vi "DNL_INL.vi"(8 "error in (no error)":errorcluster caption="错误输入（无错误）", 11 "采集信号输入":waveform(dbl)[](array[waveform])) -> (0 "error out":errorcluster caption="错误输出", 1 "INL - Min":ext, 2 "INL - Max":ext, 3 "DNL - Min":dbl, 4 "DNL":cluster{i32, i32, "Y[i]=X[i]*a+b":dbl[]}, 5 "DNL - Max":dbl, 6 "INL":cluster{dbl, i32, ext[]}, 7 "Transfer Curve":cluster{dbl[], i32[]}[](array[cluster]))   [LabVIEW 2019]
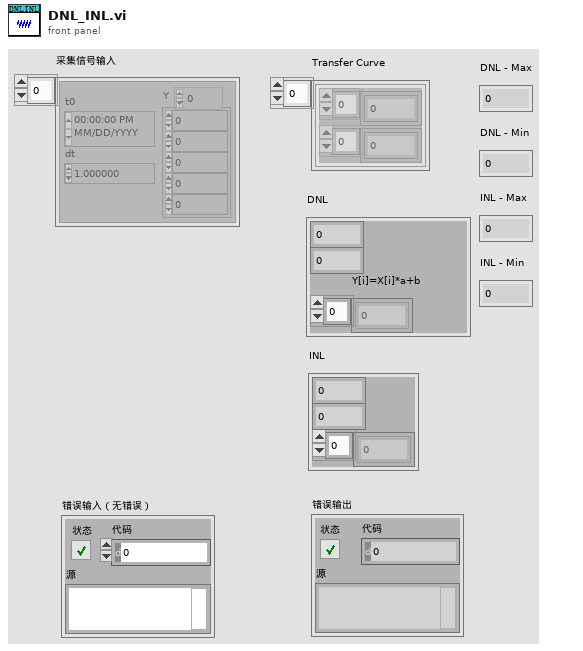
[diagram p1: front panel]
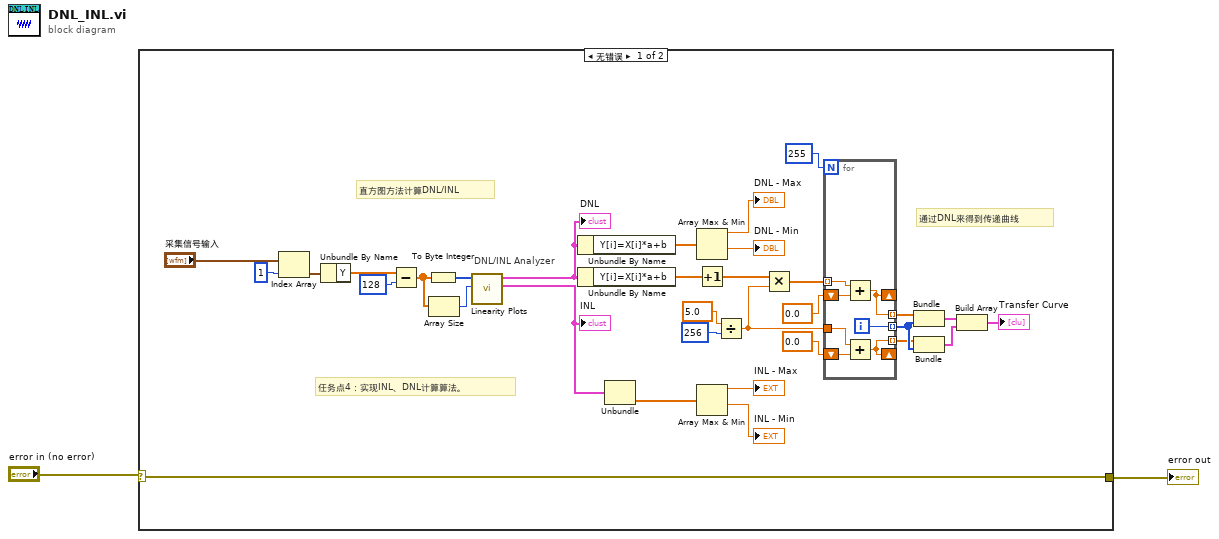
[diagram p0: block diagram]
diagram:
  n1 = case shown="无错误" "error in (no error)" {
    selector: "error in (no error)" -> [w3 w42]
    tunnel: [w3 w42] -> w1
    frame No Error {
      # "通过DNL来得到传递曲线"
      # "直方图方法计算DNL/INL"
      # "任务点4：实现INL、DNL计算算法。"
      # "DNL/INL Analyzer"
      n2 = Index Array(array="采集信号输入", index=1) -> (element=w9:waveform(dbl))
      n3 = Unbundle By Name(w9) -> ("Y"=w26:dbl[])
      n4 = Subtract(x=w26, y=128) -> (x-y=w4:dbl[])
      n5 = To Byte Integer(number=w4) -> (8bit integer=w7:i8[])
      n6 = Array Size(array=w4) -> (size(s)=w6:i32)
      n7 = call "Linearity Plots.vi"("Record length"=w6, "Waveform"=w7) -> ("INL"=w33:cluster{dbl, i32, ext[]}, "DNL"=w32:cluster{i32, i32, "Y[i]=X[i]*a+b":dbl[]})  [unwired: 7 in, 1 out]
      "INL" <- w33
      "DNL" <- w32
      n8 = Unbundle By Name(w32) -> ("Y[i]=X[i]*a+b"=w24:dbl[])
      n9 = Unbundle By Name(w32) -> ("Y[i]=X[i]*a+b"=w16:dbl[])
      n10 = Unbundle(w33) -> (w25:ext[])  [unwired: 2 out]
      n11 = Array Max & Min(array=w24) -> (max value=→"DNL - Max":dbl, min value=→"DNL - Min":dbl)  [unwired: 2 out]
      n12 = Increment(x=w16) -> (x+1=w15:dbl[])
      n13 = Array Max & Min(array=w25) -> (max value=→"INL - Max":ext, min value=→"INL - Min":ext)  [unwired: 2 out]
      n14 = Divide(x=5.0, y=u32 256) -> (x/y=w17:dbl)
      n15 = Multiply(x=w15, y=w17) -> (x*y=w18:dbl[])
      n16 = for {
        N: 255 -> [_]
        tunnel: w17 -> [w37]
        tunnel: [w41] -> w21 mode=indexing
        tunnel: w18 -> [w40] mode=indexing
        shift-right: [w38] -> _
        shift-left: 0.0 ("x") -> [w39]
        tunnel: [w38] -> w14 mode=indexing
        shift-right: [w35] -> _
        shift-left: 0.0 ("x") -> [w36]
        tunnel: [w35] -> w20 mode=indexing
        i -> [w41]
        n17 = Add(x=w40, y=w39) -> (x+y=w38:dbl)
        n18 = Add(x=w37, y=w36) -> (x+y=w35:dbl)
      }
      n19 = Bundle(w14, w21) -> (w22:cluster{dbl[], i32[]})  [unwired: 1 in]
      n20 = Bundle(w20, w21) -> (w23:cluster{dbl[], i32[]})  [unwired: 1 in]
      n21 = Build Array(w22, w23) -> (→"Transfer Curve":cluster{dbl[], i32[]}[])
    }
    frame Error {
    }
  }
  "error out" <- w1
